vi "SeparteErd.vi"(7 "return value":T1(array[cluster]), 11 "error out":errorcluster) -> (8 "Array":string[](array[string]), 15 "error IO":errorcluster)   [LabVIEW 2021]
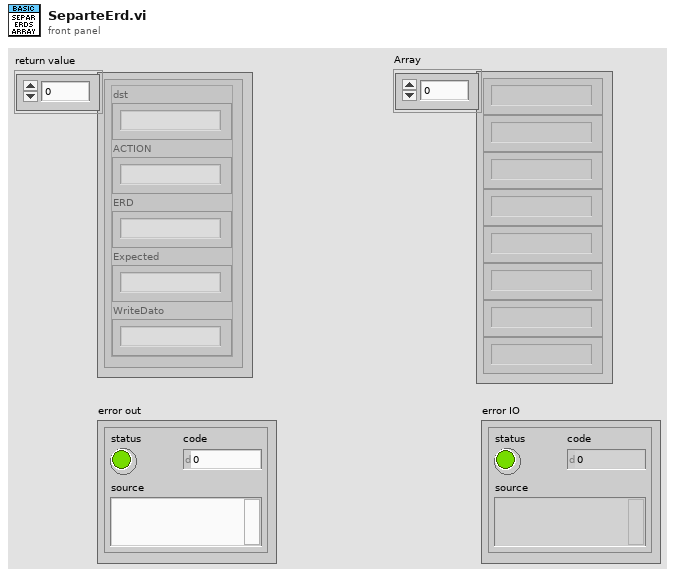
[diagram p1: front panel]
types:
  T1 = cluster{"dst":string, "ACTION":string, "ERD":string, "Expected":string, "WriteDato":string}[]
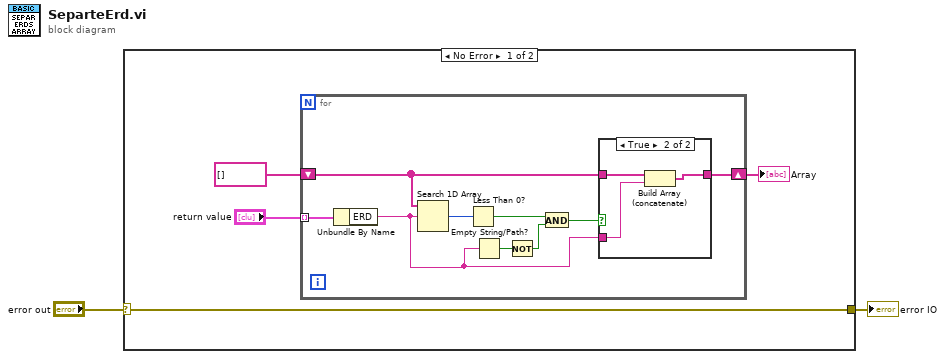
[diagram p0: block diagram]
diagram:
  n1 = case shown="No Error" "error out" {
    selector: "error out" -> [w3 w20]
    tunnel: [w3 w20] -> w1
    frame No Error {
      n2 = for {
        tunnel: "return value" -> [w15] mode=indexing
        shift-right: [w12] -> w4
        shift-left: string[] [] -> [w13]
        n3 = Unbundle By Name(w15) -> ("ERD"=w9:string)
        n4 = Search 1D Array(1D array=w13, element=w9) -> (index of element=w14:i32)  [unwired: 1 in]
        n5 = Less Than 0?(x=w14) -> (x < 0?=w11:bool)
        n6 = Empty String/Path?(string/path=w9) -> (empty?=w8:bool)
        n7 = Not(x=w8) -> (.not. x?=w7:bool)
        n8 = And(x=w11, y=w7) -> (x .and. y?=w10:bool)
        n9 = case shown="True" w10 {
          tunnel: w13 -> [w16 w19]
          tunnel: w9 -> [_ w18]
          tunnel: [w16 w17] -> w12
          frame False {
          }
          frame True {
            n10 = Build Array (concatenate)(w19, w18) -> (w17:string[])
          }
        }
      }
      "Array" <- w4
    }
    frame Error {
    }
  }
  "error IO" <- w1
